vi "SendDisplayCommand.vi"(8 "error in (no error)":errorcluster, 11 "Queue in":refnum<queue>) -> (0 "error out":errorcluster, 3 "queue out":refnum<queue>)   [LabVIEW 2016]
doc: "sends the display command to the data analyzer loop"
uses:
  DataType.ctl
  data_command_enum.ctl
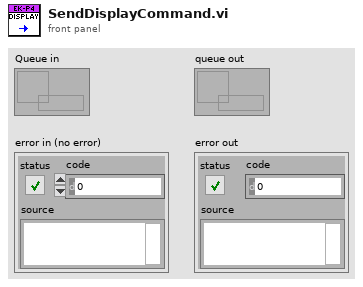
[diagram p1: front panel]
types:
  T1 = typedef "DataType.ctl" = cluster{"command":T2, "data":variant}
  T2 = typedef "data_command_enum.ctl" = enum16{"data", "display", "quit", "save", "filepath", "weak left", "state", "weak right", "strong left", "strong right", "stopRecording", "close", "sid"}
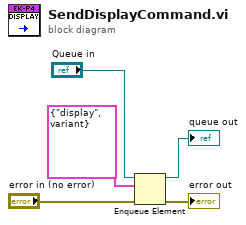
[diagram p0: block diagram]
diagram:
  n1 = Enqueue Element(queue="Queue in", element=T1 {"command"=enum."display", "data"=variant(dbl[] [])}, error in (no error)="error in (no error)") -> (queue out=→"queue out":refnum<queue>, error out=→"error out":errorcluster)  [unwired: 1 in, 1 out]
